vi "Add Global Exception Handlers.vi"(10 "Debug":bool, 11 "Exception Handler Map In":T1) -> (3 "Exception Handler Map":T1)   [LabVIEW 2020, in "HTTP Server.lvlib" / "Server.lvclass"]
uses:
  Server.lvclass
  Exception Handler Map.ctl
  Priority.ctl
  Exception Handler/Exception Handler.lvclass
  NoControllerException/NoControllerException.lvclass
  C:/dev/lv20CE/relink/lv-http-server/HTTP Server/Handler/Handler.lvclass
  C:/dev/lv20CE/relink/lv-http-server/HTTP Server/Exception Handler/Exception Handler.lvclass
  BadRequestException/BadRequestException.lvclass
  FileNotFoundException/FileNotFoundException.lvclass
  Handler/Handler.lvclass
  HTTP Server.lvlib
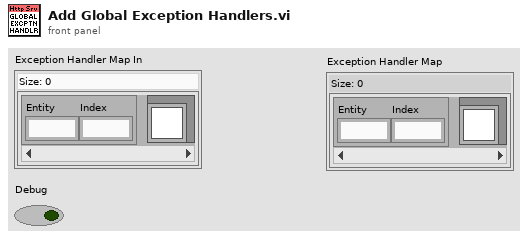
[diagram p1: front panel]
types:
  T1 = typedef "HTTP Server.lvlib/Exception Handler Map.ctl" = map{T2, refnum<class "Exception Handler.lvclass">}
  T2 = typedef "HTTP Server.lvlib/Priority.ctl" = cluster{"Entity":u16, "Index":u16}
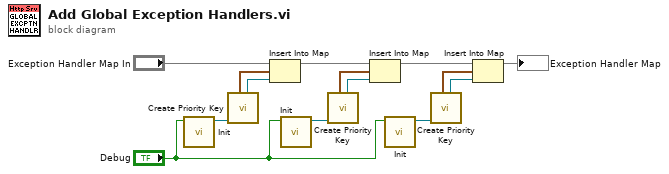
[diagram p0: block diagram]
diagram:
  n1 = call "Init.vi"("Debug"="Debug") -> ("FileNotFoundException out"=w10:refnum<class "FileNotFoundException.lvclass">)  [unwired: 9 in, 1 out]
  n2 = call "Create Priority Key.vi"("Handler In"=w10) -> ("Handler"=w12:refnum<class "FileNotFoundException.lvclass">, "Priority Key"=w13:T2)  [unwired: 8 in, 1 out]
  n3 = Insert Into Map(map in="Exception Handler Map In", key=w13, value=w12) -> (map out=w5:T1)  [unwired: 2 out]
  n4 = call "Init.vi"("Debug"="Debug") -> ("BadRequestException out"=w4:refnum<class "BadRequestException.lvclass">)  [unwired: 9 in, 1 out]
  n5 = call "Create Priority Key.vi"("Handler In"=w4) -> ("Handler"=w9:refnum<class "BadRequestException.lvclass">, "Priority Key"=w8:T2)  [unwired: 8 in, 1 out]
  n6 = Insert Into Map(map in=w5, key=w8, value=w9) -> (map out=w3:T1)  [unwired: 2 out]
  n7 = call "Init.vi"("Debug"="Debug") -> ("NoControllerException out"=w2:refnum<class "NoControllerException.lvclass">)  [unwired: 9 in, 1 out]
  n8 = call "Create Priority Key.vi"("Handler In"=w2) -> ("Handler"=w6:refnum<class "NoControllerException.lvclass">, "Priority Key"=w7:T2)  [unwired: 8 in, 1 out]
  n9 = Insert Into Map(map in=w3, key=w7, value=w6) -> (map out=→"Exception Handler Map":T1)  [unwired: 2 out]
